vi "LV to ITX  Retrieve.vi"(0 "File or Folder Path":path=path "C:/", 1 "Data Type":T1=enum."DAT", 2 "DAT header length":i32=11, 5 "offset":i32, 7 "length":i32=1, 9 "index":T2={"A"=1, "B"=0, "C"=2, "D"=0, "E"=3, "N1"=0, "N2"=0, "N3"=0, "N4"=0}, 11 "error in (no error)":errorcluster) -> (4 "A vs B":cluster{dbl[], dbl[]}[](graph), 6 "C vs D":cluster{dbl[], dbl[]}[](graph), 8 "E":dbl[][](graph), 10 "N":cluster{"N1":dbl, "N2":dbl, "N3":dbl, "N4":dbl}={"N1"=0.0624995231628418, "N2"=0.0624995231628418, "N3"=0.0624995231628418, "N4"=0.0624995231628418} {"N4" format="%#_6p"; "N3" format="%#_6p"; "N2" format="%#_6p"; "N1" format="%#_6p"}, 14 "Comments":string)   [LabVIEW 2016, in "LV to ITX.lvclass"]
uses:
  LV to ITX.lvclass
  <vilib>/Utility/miscctls.llb/LVOffsetAndMultiplierTypeDef.ctl
  Typedefs/Retrieve Data Type.ctl
  <userlib>/LevyLab/Graph Utilities/graph_utilities.lvclass
panel:
  in  "D  is time?":bool
  in  "B is time?":bool
  out "time":string[][](table)
  in  "Use Folder Index File?":bool
  in  "Generate Folder Index File?":bool
  in  "Ez name":string="Ez name"
  in  "Ey name":string="Ey name"
  in  "Ex name":string="Ex name"
  in  "C y name":string="C y name"
  in  "D x name":string="D x name"
  in  "A y name":string="A y name"
  in  "B x name":string="B x name"
  out "Index, Wavenames":string[][](table)
  in  "recolor traces?":bool
  in  "Ex":T3={"Offset"=0.0, "Multiplier"=1.0}
  in  "Ey":T3={"Offset"=0.0, "Multiplier"=1.0}
  out "Path":path
  out "counter":i32
  out "pattern":string="*.dat"
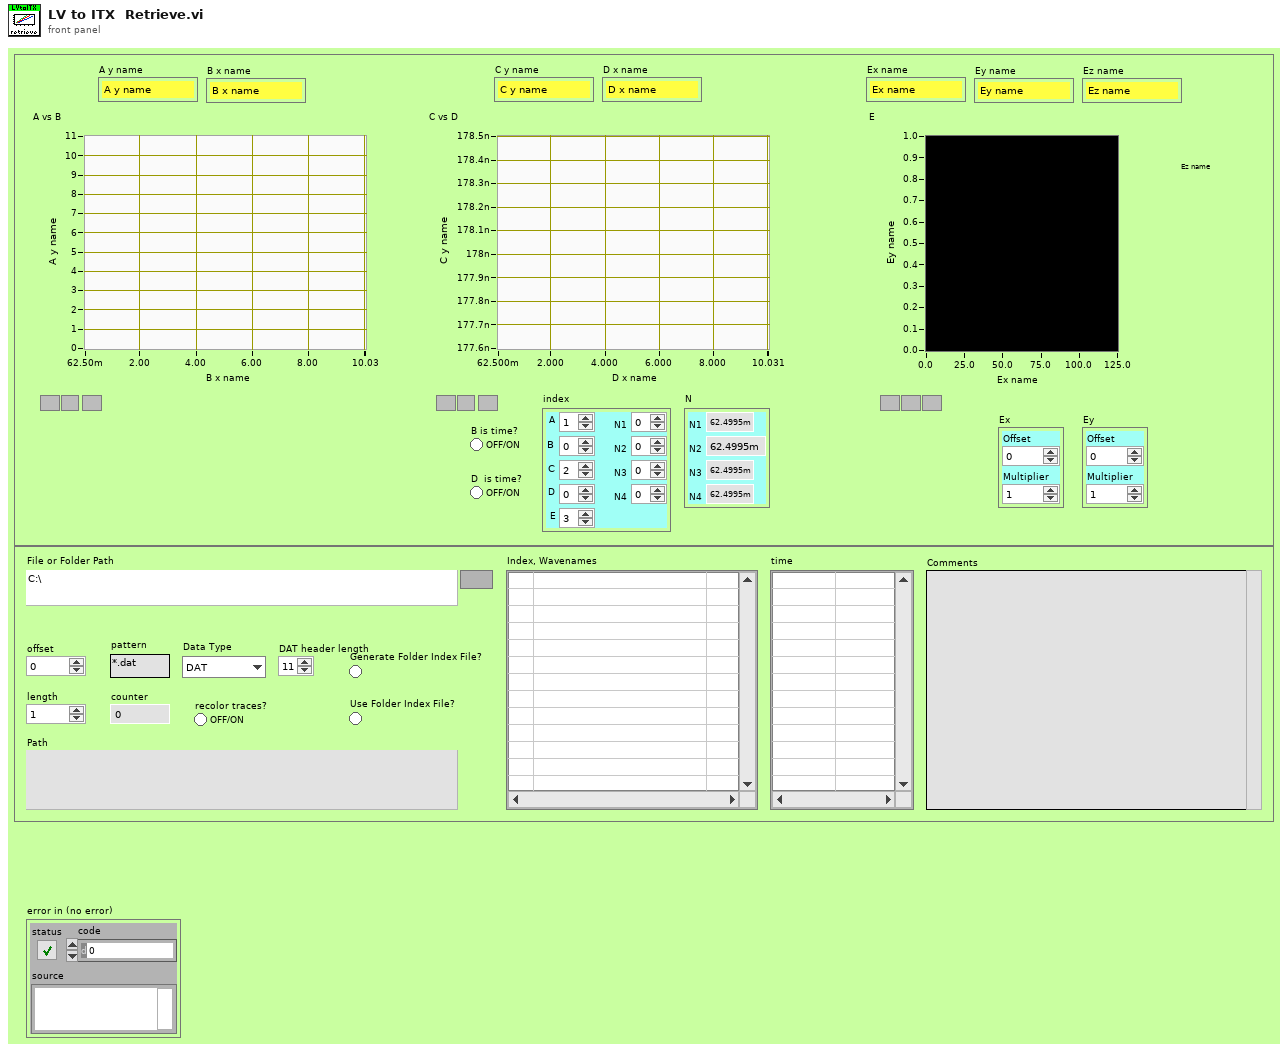
[diagram p1: front panel]
types:
  T1 = typedef "LV to ITX.lvclass/Retrieve Data Type.ctl" = enum16{"ITX", "ITX w/ 2D", "DAT", "TDMS"}
  T2 = cluster{"A":i32, "B":i32, "C":i32, "D":i32, "E":i32, "N1":i32, "N2":i32, "N3":i32, "N4":i32}
  T3 = typedef "LVOffsetAndMultiplierTypeDef.ctl" = cluster{"Offset":dbl, "Multiplier":dbl}
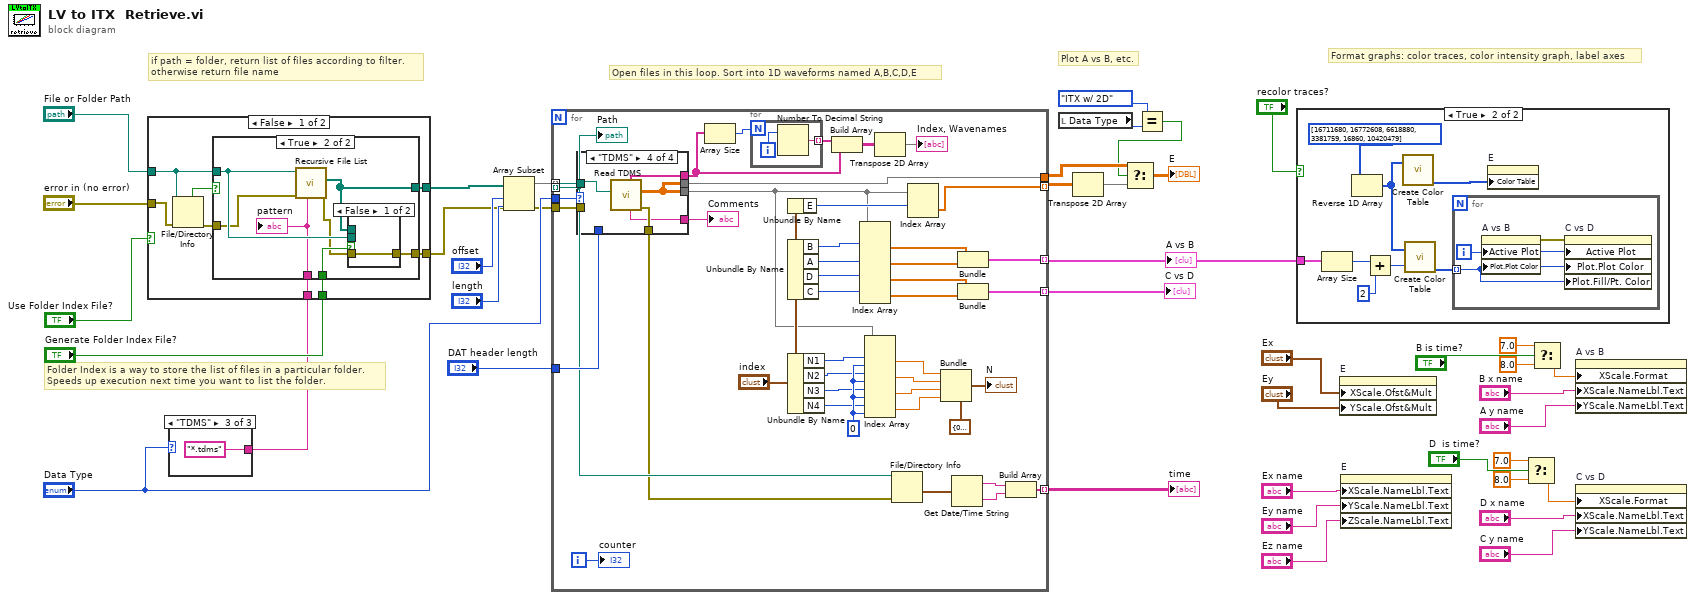
[diagram p0: block diagram]
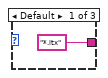
[diagram p2: hidden frame]
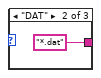
[diagram p3: hidden frame]
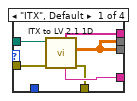
[diagram p5: hidden frame]
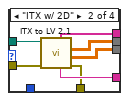
[diagram p6: hidden frame]
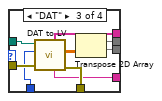
[diagram p7: hidden frame]
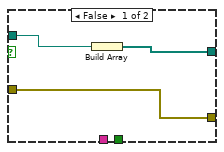
[diagram p8: hidden frame]
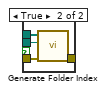
[diagram p9: hidden frame]
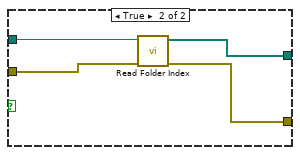
[diagram p10: hidden frame]
diagram:
  # "Plot A vs B, etc."
  # "Format graphs: color traces, color intensity graph, label axes"
  # "Open files in this loop. Sort into 1D waveforms named A,B,C,D,E"
  # "Folder Index is a way to store the list of files in a particular folder.\nSpeeds up execution next time you want to list the folder."
  # "if path = folder, return list of files according to filter.\notherwise return file name"
  n1 = case shown="\"TDMS\"" "Data Type" {
    tunnel: ["*.itx" ("pattern") "*.dat" ("pattern") "*.tdms" ("pattern")] -> w4
    frame Default {
    }
    frame "DAT" {
    }
    frame "TDMS" {
    }
  }
  n2 = case shown="False" "Use Folder Index File?" {
    tunnel: [w49 w69] -> w38
    tunnel: "File or Folder Path" -> [w51 w70]
    tunnel: "Generate Folder Index File?" -> [w48 _]
    tunnel: w4 -> [w47 _]
    tunnel: "error in (no error)" -> [w46 w68]
    tunnel: [w44 w67] -> w1
    frame False {
      n3 = File/Directory Info(path=w51, error in=w46) -> (directory=w50:bool, error out=w45:errorcluster)  [unwired: 5 out]
      n4 = case shown="True" w50 {
        tunnel: [w54 w60] -> w49
        tunnel: w51 -> [w53 w61]
        tunnel: w48 -> [_ w57]
        tunnel: w47 -> [_ w59]
        tunnel: w45 -> [w52 w58]
        tunnel: [w52 w55] -> w44
        frame False {
          n5 = Build Array(w53) -> (w54:path[])
        }
        frame True {
          n6 = call <vilib>:"Recursive File List.vi"("pattern"=w59, "error in (no error)"=w58, "Folder Path"=w61) -> ("error out"=w56:errorcluster, "All Files in Dir"=w60:path[])  [unwired: 4 in, 3 out]
          n7 = case shown="False" w57 {
            tunnel: w60 -> [_ w66]
            tunnel: w61 -> [_ w65]
            tunnel: w56 -> [w62 w64]
            tunnel: [w62 w63] -> w55
            frame False {
            }
            frame True {
              n8 = call "Generate Folder Index.vi"("error in (no error)"=w64, "File or Folder Path"=w65, "All Files in Dir"=w66) -> ("error out"=w63:errorcluster)  [unwired: 8 in]
            }
          }
          "pattern" <- w59
        }
      }
    }
    frame True {
      n9 = call "Read Folder Index.vi"("error in (no error)"=w68, "File or Folder Path"=w70) -> ("error out"=w67:errorcluster, "Files"=w69:path[])  [unwired: 8 in]
    }
  }
  n10 = Array Subset(array=w38, index="offset", length="length") -> (w17:path[])
  n11 = for {
    tunnel: w17 -> [w76] mode=indexing
    tunnel: [w76] -> _ mode=indexing
    tunnel: [w110] -> w29 mode=indexing
    tunnel: [w109] -> w28 mode=indexing
    tunnel: [w88] -> w33 mode=indexing
    tunnel: [w102] -> w31
    tunnel: [w80] -> w20 mode=indexing
    tunnel: "Data Type" -> [w78]
    tunnel: "DAT header length" -> [w77]
    tunnel: w1 -> [w75]
    i -> [w112]
    w101 = 0 ("disabled index (col)")
    n12 = case shown="\"TDMS\"" w78 {
      tunnel: [w119 w126 w128 w136] -> w111
      tunnel: [w116 w123 w134 w139] -> w81
      tunnel: w76 -> [w120 w127 w135 w140]
      tunnel: [w115 w121 w129 w138] -> w103
      tunnel: [w116 w122 w134 w139] -> w102
      tunnel: w77 -> [_ _ w130 _]
      tunnel: w75 -> [w118 w124 w133 _]
      tunnel: [w117 w125 w132 w137] -> w74
      frame "ITX", Default {
        n13 = call "ITX to LV 2.1 1D.vi"("error in"=w118, "file (use dialog)"=w120) -> ("error out"=w117:errorcluster, "1D arrays"=w116:dbl[][], "Notes"=w119:string, "base wavenames"=w115:string[])  [unwired: 4 in, 2 out]
      }
      frame "ITX w/ 2D" {
        n14 = call "ITX to LV 2.1.vi"("error in"=w124, "file (use dialog)"=w127) -> ("error out"=w125:errorcluster, "1D arrays"=w123:dbl[][], "2D array"=w122:dbl[][], "Notes"=w126:string, "wave names"=w121:string[])  [unwired: 3 in, 2 out]
      }
      frame "DAT" {
        n15 = call "DAT to LV.vi"("error in (no error)"=w133, "header length"=w130, "File Path"=w135) -> ("error out"=w132:errorcluster, "Data"=w131:dbl[][], "Comments"=w128:string, "Wavenames"=w129:string[])  [unwired: 4 in, 1 out]
        n16 = Transpose 2D Array(2D array=w131) -> (transposed array=w134:dbl[][])
      }
      frame "TDMS" {
        n17 = call "Read TDMS.vi"("path"=w140) -> ("error out"=w137:errorcluster, "Data"=w139:dbl[][], "Comments"=w136:string, "Wavenames"=w138:string[])  [unwired: 4 in, 3 out]
      }
    }
    "Comments" <- w111
    n18 = Array Size(array=w103) -> (size(s)=w71:i32)
    n19 = for {
      N: w71 -> [_]
      tunnel: [w113] -> w107 mode=indexing
      i -> [w114]
      n20 = Number To Decimal String(number=w114) -> (decimal integer string=w113:string)  [unwired: 1 in]
    }
    n21 = Unbundle By Name("index") -> ("E"=w93:i32)
    n22 = Unbundle By Name("index") -> ("B"=w92:i32, "A"=w91:i32, "D"=w90:i32, "C"=w89:i32)
    n23 = Unbundle By Name("index") -> ("N1"=w94:i32, "N2"=w95:i32, "N3"=w96:i32, "N4"=w97:i32)
    n24 = Build Array(w107, w103) -> (w104:string[][])
    n25 = Index Array(array=w81, index (row) #1=w92, index (row) #2=w91, index (row) #3=w90, index (row) #4=w89) -> (element #1=w86:dbl[], element #2=w85:dbl[], element #3=w105:dbl[], element #4=w108:dbl[])  [unwired: 4 in]
    n26 = Index Array(array=w81, index (row) #1=w94, index (col) #1=w101, index (row) #2=w95, index (col) #2=w101, index (row) #3=w96, index (col) #3=w101, index (row) #4=w97, index (col) #4=w101) -> (element #1=w82:dbl, element #2=w83:dbl, element #3=w84:dbl, element #4=w100:dbl)
    n27 = Transpose 2D Array(2D array=w104) -> (transposed array=→"Index, Wavenames":string[][])
    n28 = File/Directory Info(path=w76, error in=w74) -> (last mod=w79:timestamp)  [unwired: 6 out]
    n29 = Index Array(array=w81, index (row)=w93) -> (element=w88:dbl[])  [unwired: 1 in]
    n30 = Bundle(cluster=cluster{"N1":dbl, "N2":dbl, "N3":dbl, "N4":dbl} {"N1"=0.0, "N2"=0.0, "N3"=0.0, "N4"=0.0}, "N1"=w82, "N2"=w83, "N3"=w84, "N4"=w100) -> (→"N":cluster{"N1":dbl, "N2":dbl, "N3":dbl, "N4":dbl})
    n31 = Get Date/Time String(seconds (now)=w79) -> (date string=w72:string, time string=w73:string)  [unwired: 2 in]
    n32 = Bundle("Data"=w86, "Data"=w85) -> (w110:cluster{"Data":dbl[], "Data":dbl[]})  [unwired: 1 in]
    n33 = Bundle("Data"=w105, "Data"=w108) -> (w109:cluster{"Data":dbl[], "Data":dbl[]})  [unwired: 1 in]
    n34 = Build Array(w72, w73) -> (w80:string[])
    "counter" <- w112
    "Path" <- w76
  }
  "A vs B" <- w29
  "C vs D" <- w28
  "time" <- w20
  n35 = local read "Data Type"() -> (w7:T1)
  n36 = Transpose 2D Array(2D array=w33) -> (transposed array=w34:dbl[][])
  n37 = Equal?(x=enum16{"ITX", "ITX w/ 2D", "DAT"}."ITX w/ 2D" ("Enum"), y=w7) -> (x = y?=w5:bool)
  n38 = Select(t=w31, s=w5, f=w34) -> (s? t:f=→"E":dbl[][])
  n39 = case shown="True" "recolor traces?" {
    tunnel: w29 -> [_ w143]
    frame False {
    }
    frame True {
      n40 = Array Size(array=w143) -> (size(s)=w144:i32)
      n41 = Reverse 1D Array(array=u32[] [16711680, 16772608, 6618880, 3381759, 16860, 10420479] ("color scale")) -> (reversed array=w142:u32[])
      n42 = Add(x=w144, y=2 ("x")) -> (x+y=w148:i32)
      n43 = call <userlib>:"Create Color Table.vi"("Colors []"=w142) -> ("Color Tbl"=w146:u32[])  [unwired: 1 in, 3 out]
      n44 = call <userlib>:"Create Color Table.vi"("Colors []"=w142, "Size (256)"=w148) -> ("Color Tbl"=w145:u32[])  [unwired: 3 out]
      n45 = for {
        tunnel: w145 -> [w149] mode=indexing
        i -> [w150]
        n46 = property on="A vs B" class="XYGraph (strict)"("Active Plot"=w150, "Plot.Plot Color"=w149) -> (error out=w151:errorcluster)  [unwired: 2 in, 1 out]
        n47 = property on="C vs D" class="XYGraph (strict)"(error in=w151, "Active Plot"=w150, "Plot.Plot Color"=w149, "Plot.Fill/Pt. Color"=w149) -> ()  [unwired: 1 in, 2 out]
      }
      n48 = property on="E" class="IntGraph (strict)"("Color Table"=w146) -> ()  [unwired: 2 in, 2 out]
    }
  }
  n49 = property on="E" class="IntGraph (strict)"("XScale.Ofst&Mult"="Ex", "YScale.Ofst&Mult"="Ey") -> ()  [unwired: 2 in, 2 out]
  n50 = property on="E" class="IntGraph (strict)"("XScale.NameLbl.Text"="Ex name", "YScale.NameLbl.Text"="Ey name", "ZScale.NameLbl.Text"="Ez name") -> ()  [unwired: 2 in, 2 out]
  n51 = Select(t=7.0, s="D  is time?", f=8.0) -> (s? t:f=w13:dbl)
  n52 = Select(t=7.0, s="B is time?", f=8.0) -> (s? t:f=w14:dbl)
  n53 = property on="A vs B" class="XYGraph (strict)"("XScale.Format"=w14, "XScale.NameLbl.Text"="B x name", "YScale.NameLbl.Text"="A y name") -> ()  [unwired: 2 in, 2 out]
  n54 = property on="C vs D" class="XYGraph (strict)"("XScale.Format"=w13, "XScale.NameLbl.Text"="D x name", "YScale.NameLbl.Text"="C y name") -> ()  [unwired: 2 in, 2 out]
